vi "HEWH Flow Data.vi"(8 "error in (no error)":errorcluster, 10 "Laurel IP Address Cold in":string, 11 "Laurel IP Address Hot":string) -> (0 "error out":errorcluster, 1 "Flow Selector":T1, 2 "Gallons":dbl, 3 "Flow Rate":dbl, 4 "Emerson Flow Meter Data Output":T2)   [LabVIEW 2019]
uses:
  Drivers/Emerson 5700 Transmitter/Type Definitions/Emerson 5700 Data.ctl
  Type Definitions/Flow Meter Selector.ctl
  Drivers/Laurel Meter/Type Definitions/Laurel Serial Commands.ctl
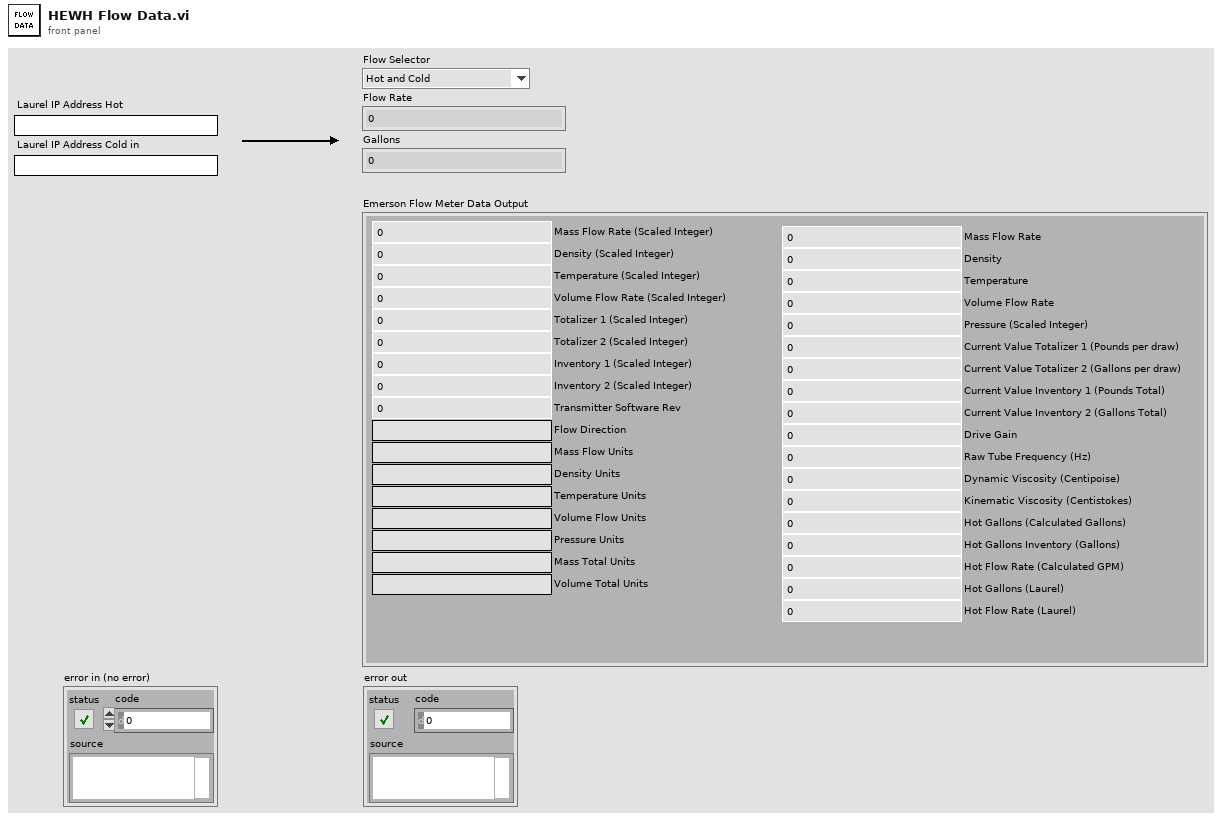
[diagram p1: front panel]
types:
  T1 = typedef "Flow Meter Selector.ctl" = enum16{"Hot and Cold", "Hot", "Cold", "None"}
  T2 = typedef "Emerson 5700 Data.ctl" = cluster{"Mass Flow Rate (Scaled Integer)":u16, "Density (Scaled Integer)":u16, "Temperature (Scaled Integer)":u16, "Volume Flow Rate (Scaled Integer)":u16, "Totalizer 1 (Scaled Integer)":u16, "Totalizer 2 (Scaled Integer)":u16, "Transmitter Software Rev":u16, "Flow Direction":string, "Mass Flow Units":string, "Density Units":string, "Temperature Units":string, "Volume Flow Units":string, "Pressure Units":string, "Mass Total Units":string, "Volume Total Units":string, "Inventory 1 (Scaled Integer)":u16, "Inventory 2 (Scaled Integer)":u16, "Mass Flow Rate":dbl, "Density":dbl, "Temperature":dbl, "Volume Flow Rate":dbl, "Pressure (Scaled Integer)":u16, "Current Value Totalizer 1 (Pounds per draw)":dbl, "Current Value Totalizer 2 (Gallons per draw)":dbl, "Current Value Inventory 1 (Pounds Total)":dbl, "Current Value Inventory 2 (Gallons Total)":dbl, "Drive Gain":dbl, "Raw Tube Frequency (Hz)":dbl, "Dynamic Viscosity (Centipoise)":dbl, "Kinematic Viscosity (Centistokes)":dbl, "Hot Gallons (Calculated Gallons)":dbl, "Hot Flow Rate (Calculated GPM)":dbl, "Hot Gallons Inventory (Gallons)":dbl, "Hot Flow Rate (Laurel)":dbl, "Hot Gallons (Laurel)":dbl}
  T3 = typedef "Laurel Serial Commands.ctl" = string
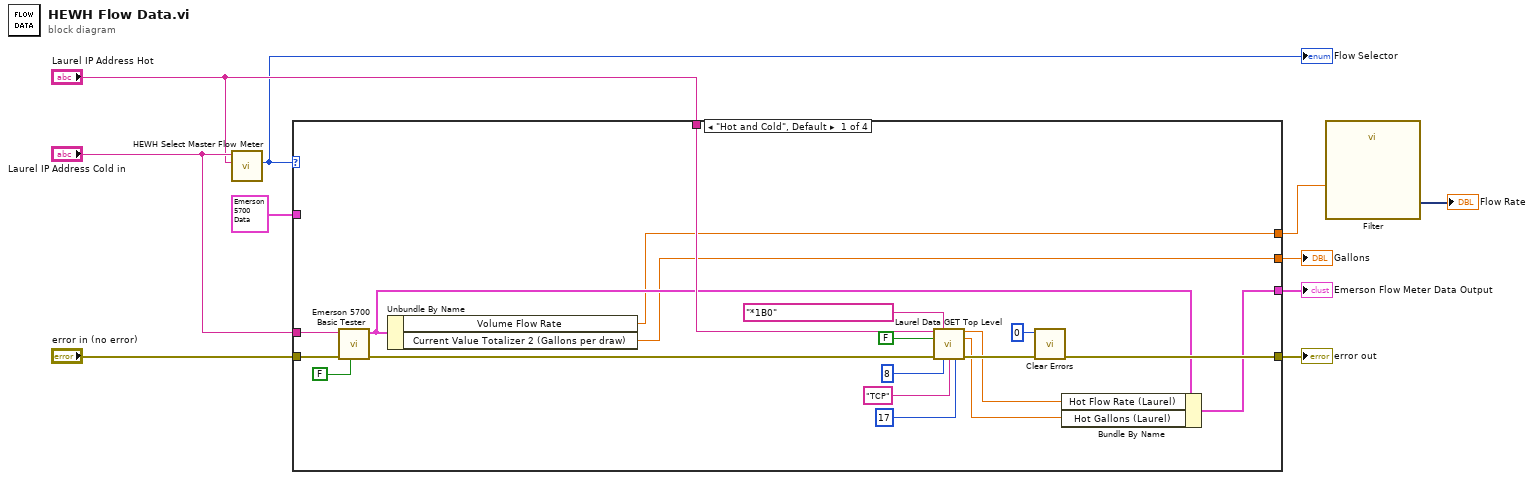
[diagram p0: block diagram]
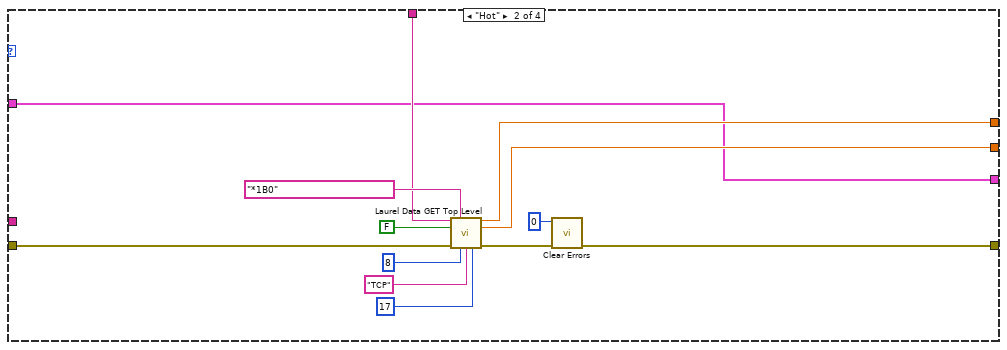
[diagram p2: hidden frame]
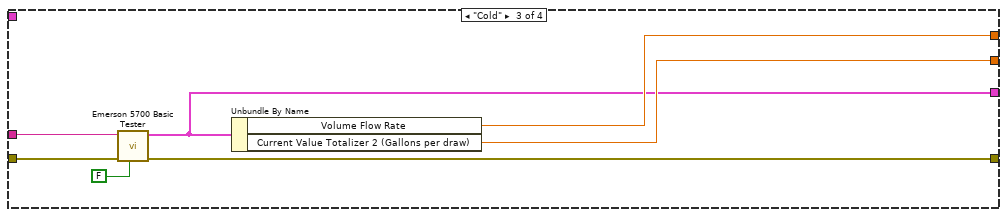
[diagram p3: hidden frame]
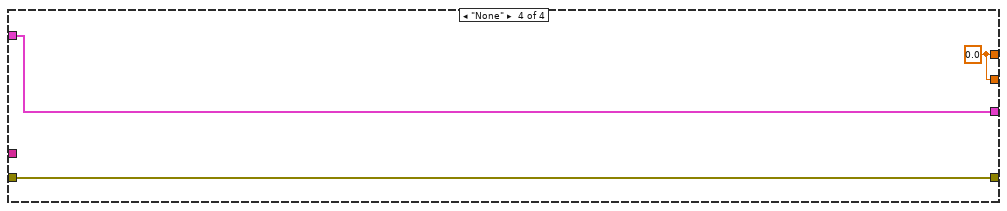
[diagram p4: hidden frame]
diagram:
  n1 = call "HEWH Select Master Flow Meter.vi"("Laurel Hot IP Address"="Laurel IP Address Hot", "Laurel Cold IP Address"="Laurel IP Address Cold in") -> ("Flow Selector"=w5:T1)  [unwired: 7 in, 2 out]
  "Flow Selector" <- w5
  n2 = case shown="\"Hot and Cold\", Default" w5 {
    tunnel: "error in (no error)" -> [w29 w35 w48 w50]
    tunnel: "Laurel IP Address Cold in" -> [w28 _ w47 _]
    tunnel: "Laurel IP Address Hot" -> [w27 w34 _ _]
    tunnel: [w25 w33 w44 w50] -> w9
    tunnel: [w15 w30 w43 w51] -> w8
    tunnel: [w14 w32 w46 w52] -> w2
    tunnel: [w13 w31 w45 w52] -> w4
    tunnel: T2 {"Mass Flow Rate (Scaled Integer)"=0, "Density (Scaled Integer)"=0, "Temperature (Scaled Integer)"=0, "Volume Flow Rate (Scaled Integer)"=0, "Totalizer 1 (Scaled Integer)"=0, "Totalizer 2 (Scaled Integer)"=0, "Transmitter Software Rev"=0, "Flow Direction"="", "Mass Flow Units"="", "Density Units"="", "Temperature Units"="", "Volume Flow Units"="", "Pressure Units"="", "Mass Total Units"="", "Volume Total Units"="", "Inventory 1 (Scaled Integer)"=0, "Inventory 2 (Scaled Integer)"=0, "Mass Flow Rate"=0.0, "Density"=0.0, "Temperature"=0.0, "Volume Flow Rate"=0.0, "Pressure (Scaled Integer)"=0, "Current Value Totalizer 1 (Pounds per draw)"=0.0, "Current Value Totalizer 2 (Gallons per draw)"=0.0, "Current Value Inventory 1 (Pounds Total)"=0.0, "Current Value Inventory 2 (Gallons Total)"=0.0, "Drive Gain"=0.0, "Raw Tube Frequency (Hz)"=0.0, "Dynamic Viscosity (Centipoise)"=0.0, "Kinematic Viscosity (Centistokes)"=0.0, "Hot Gallons (Calculated Gallons)"=0.0, "Hot Flow Rate (Calculated GPM)"=0.0, "Hot Gallons Inventory (Gallons)"=0.0, "Hot Flow Rate (Laurel)"=0.0, "Hot Gallons (Laurel)"=0.0} ("Emerson Flow Meter Data Output") -> [_ w30 _ w51]
    frame "Hot and Cold", Default {
      n3 = call "Emerson 5700 Basic Tester.vi"("Check for Emerson?"=FALSE, "Error In"=w29, "Remote IP Address"=w28) -> ("Error Out"=w26:errorcluster, "Emerson Flow Meter Data Output"=w16:T2)  [unwired: 7 in]
      n4 = Unbundle By Name(w16) -> ("Volume Flow Rate"=w14:dbl, "Current Value Totalizer 2 (Gallons per draw)"=w13:dbl)
      n5 = call "Laurel Data GET Top Level.vi"("Laurel IP Address"=w27, "Laurel Serial Commands"=T3 "*1B0", "Use Delay"=FALSE, "error in (no error)"=w26, "byte count"=8, "Laurel Communication Type"="TCP", "All Items Byte Count (Flow Rate)"=17 ("byte count")) -> ("Flow Rate (Item 1)"=w12:dbl, "Gallons (Item 2)"=w11:dbl, "error out"=w18:errorcluster)  [unwired: 3 in, 3 out]
      n6 = call <vilib>:"Clear Errors.vi"("error in (no error)"=w18, "specific error code to clear (0: all)"=0) -> ("error out"=w25:errorcluster)  [unwired: 4 in, 1 out]
      n7 = Bundle By Name(cluster=w16, "Hot Flow Rate (Laurel)"=w12, "Hot Gallons (Laurel)"=w11) -> (w15:T2)
    }
    frame "Hot" {
      n8 = call "Laurel Data GET Top Level.vi"("Laurel IP Address"=w34, "Laurel Serial Commands"=T3 "*1B0", "Use Delay"=FALSE, "error in (no error)"=w35, "byte count"=8, "Laurel Communication Type"="TCP", "All Items Byte Count (Flow Rate)"=17 ("byte count")) -> ("Flow Rate (Item 1)"=w32:dbl, "Gallons (Item 2)"=w31:dbl, "error out"=w37:errorcluster)  [unwired: 3 in, 3 out]
      n9 = call <vilib>:"Clear Errors.vi"("error in (no error)"=w37, "specific error code to clear (0: all)"=0) -> ("error out"=w33:errorcluster)  [unwired: 4 in, 1 out]
    }
    frame "Cold" {
      n10 = call "Emerson 5700 Basic Tester.vi"("Check for Emerson?"=FALSE, "Error In"=w48, "Remote IP Address"=w47) -> ("Error Out"=w44:errorcluster, "Emerson Flow Meter Data Output"=w43:T2)  [unwired: 7 in]
      n11 = Unbundle By Name(w43) -> ("Volume Flow Rate"=w46:dbl, "Current Value Totalizer 2 (Gallons per draw)"=w45:dbl)
    }
    frame "None" {
      w52 = 0.0 ("Volume Flow Rate")
    }
  }
  "Emerson Flow Meter Data Output" <- w8
  "error out" <- w9
  "Gallons" <- w4
  n12 = call "Filter"("Signal"=w2) -> ("Filtered Signal"=→"Flow Rate":dynamicdata)  [unwired: 9 in, 1 out]
